vi "XML_ControlConfig.vi"(8 "error in (no error)":errorcluster, 9 "Save?(T)":bool=TRUE) -> (0 "error out":errorcluster)   [LabVIEW 2012]
uses:
  <vilib>/Utility/xml.llb/Read From XML File(array).vi
  <vilib>/Utility/xml.llb/Write to XML File(array).vi
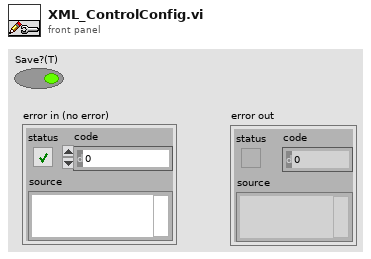
[diagram p1: front panel]
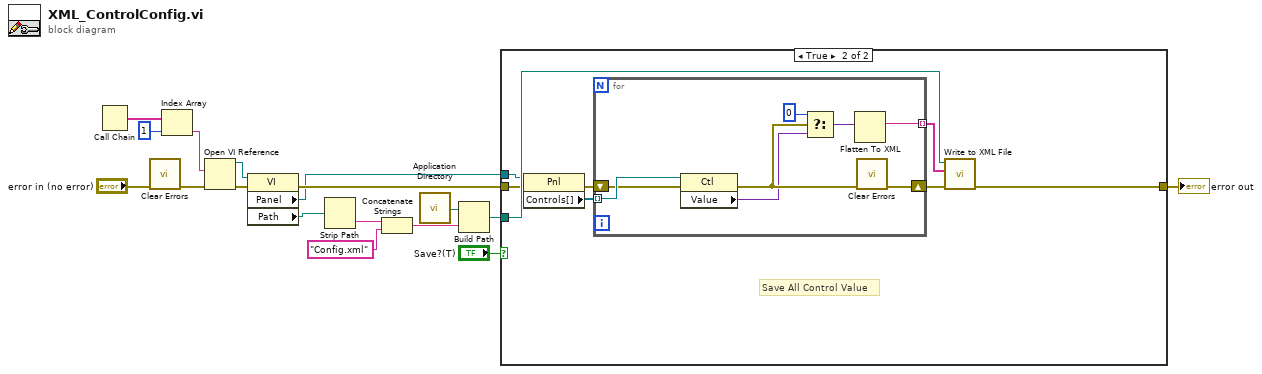
[diagram p0: block diagram]
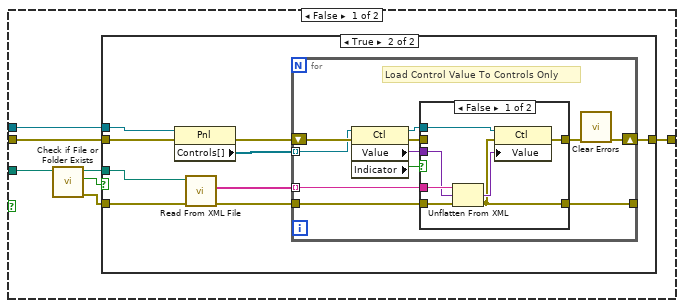
[diagram p2: hidden frame]
diagram:
  n1 = Call Chain() -> (call chain=w13:string[])
  n2 = call <vilib>:"Clear Errors.vi"("error in (no error)"="error in (no error)") -> ("error out"=w1:errorcluster)  [unwired: 6 in]
  n3 = Index Array(array=w13, index=1) -> (element=w11:string)
  n4 = Open VI Reference(vi path=w11, error in (no error)=w1) -> (vi reference=w10:refnum<vi>, error out=w4:errorcluster)  [unwired: 4 in]
  n5 = property class="VI"(reference=w10, error in=w4) -> (error out=w15:errorcluster, "Panel"=w14:refnum<vi>, "Path"=w9:path)  [unwired: 1 out]
  n6 = Strip Path(path=w9) -> (name=w7:string)  [unwired: 1 out]
  n7 = Concatenate Strings(w7, "Config.xml" ("string")) -> (w6:string)
  n8 = call <vilib>:"Application Directory.vi"() -> ("Application Directory"=w8:path)
  n9 = Build Path(base path=w8, name or relative path=w6) -> (appended path=w17:path)
  n10 = case shown="True" "Save?(T)" {
    tunnel: w17 -> [w24 w58]
    tunnel: [w20 w55] -> w16
    tunnel: w15 -> [w18 w56]
    tunnel: w14 -> [w19 w57]
    frame False {
      n11 = call <vilib>:"Check if File or Folder Exists.vi"("path"=w24) -> ("error out"=w21:errorcluster, "file or folder exists?"=w23:bool, "dup path"=w22:path)  [unwired: 8 in]
      n12 = case shown="True" w23 {
        tunnel: w22 -> [_ w34]
        tunnel: w21 -> [_ w33]
        tunnel: [w25 w29] -> w20
        tunnel: w19 -> [_ w30]
        tunnel: w18 -> [w25 w27]
        frame False {
        }
        frame True {
          n13 = property class="Pnl"(reference=w30, error in=w27) -> (error out=w32:errorcluster, "Controls[]"=w31:refnum<vi>[])  [unwired: 1 out]
          n14 = call-poly <vilib>:"Read From XML File.vi"("error in (no error)"=w33, "XML File Path"=w34) -> ("error out"=w26:errorcluster, "XML Elements"=w28:string[])  [unwired: 7 in, 1 out]
          n15 = for {
            tunnel: w31 -> [w40] mode=indexing
            shift-right: [w44] -> w29
            shift-left: w32 -> [w41]
            tunnel: w28 -> [w43] mode=indexing
            tunnel: w26 -> [w37]
            tunnel: [w36] -> _
            # "Load Control Value To Controls Only"
            n16 = property class="Ctl"(reference=w40, error in=w41) -> (reference out=w39:refnum<vi>, error out=w38:errorcluster, "Value"=w42:variant, "Indicator"=w35:bool)
            n17 = case shown="False" w35 {
              tunnel: [w52 w54] -> w45
              tunnel: w43 -> [w51 _]
              tunnel: w42 -> [w49 _]
              tunnel: w39 -> [w48 _]
              tunnel: w38 -> [_ w54]
              tunnel: w37 -> [w47 w53]
              tunnel: [w46 w53] -> w36
              frame False {
                n18 = Unflatten From XML(xml string=w51, type=w49, error in (no error)=w47) -> (value=w50:variant, error out=w46:errorcluster)
                n19 = property class="Ctl"(reference=w48, error in=w46, "Value"=w50) -> (error out=w52:errorcluster)  [unwired: 1 out]
              }
              frame True {
                # "ignore indicator"
              }
            }
            n20 = call <vilib>:"Clear Errors.vi"("error in (no error)"=w45) -> ("error out"=w44:errorcluster)  [unwired: 6 in]
          }
        }
      }
    }
    frame True {
      # "Save All Control Value"
      n21 = property class="Pnl"(reference=w57, error in=w56) -> (error out=w60:errorcluster, "Controls[]"=w59:refnum<vi>[])  [unwired: 1 out]
      n22 = for {
        tunnel: w59 -> [w70] mode=indexing
        shift-right: [w68] -> w61
        shift-left: w60 -> [w69]
        tunnel: [w63] -> w62 mode=indexing
        n23 = property class="Ctl"(reference=w70, error in=w69) -> (error out=w67:errorcluster, "Value"=w65:variant)  [unwired: 1 out]
        n24 = Select(t=0, s=w67, f=w65) -> (s? t:f=w64:variant)
        n25 = Flatten To XML(anything=w64) -> (xml string=w63:string)
        n26 = call <vilib>:"Clear Errors.vi"("error in (no error)"=w67) -> ("error out"=w68:errorcluster)  [unwired: 6 in]
      }
      n27 = call-poly <vilib>:"Write to XML File.vi"("error in (no error)"=w61, "XML Input"=w62, "XML File Path"=w58) -> ("error out"=w55:errorcluster)  [unwired: 6 in, 2 out]
    }
  }
  "error out" <- w16
